vi "setUp.vi"(8 "error in (no error)":errorcluster, 11 "reference in":refnum<class "Test TCP Stream Disconnect.lvclass">) -> (0 "error out":errorcluster, 3 "reference out":refnum<class "Test TCP Stream Disconnect.lvclass">)   [LabVIEW 2020, in "Test TCP Stream Disconnect.lvclass"]
doc: "setUp runs prior to the test method during test execution. Use this method to initialize any object data required by your tests."
uses:
  Test TCP Stream Disconnect.lvclass
  <vilib>/addons/_JKI Toolkits/VI Tester/TestCase.llb/TestCase.lvclass
  Source/Protocols/TCP Strategy/TCP Stream Initiator/TCP Stream Initiator.lvclass
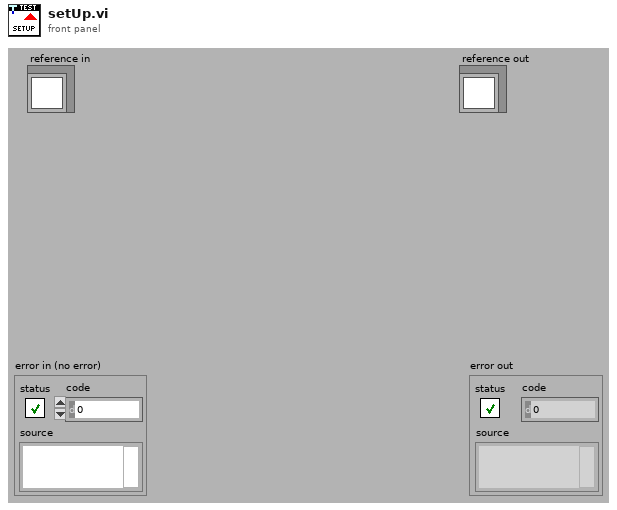
[diagram p1: front panel]
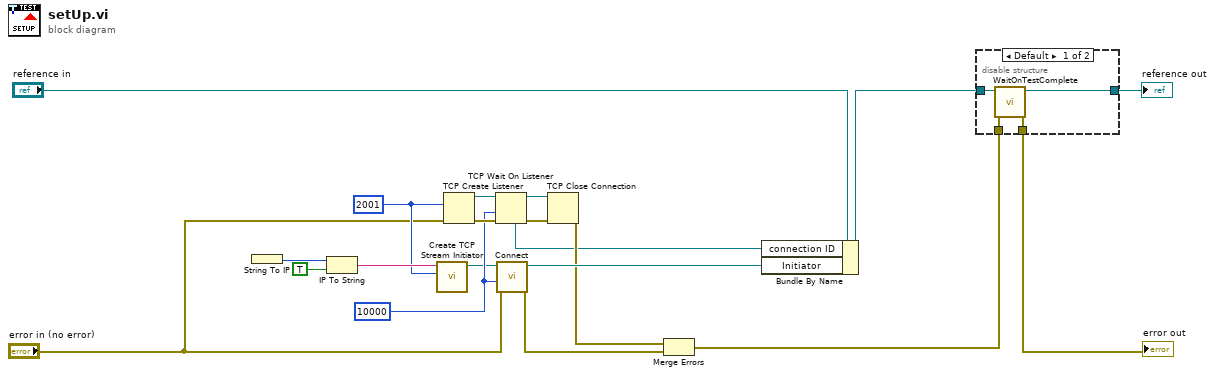
[diagram p0: block diagram]
diagram:
  w7 = u16 2001 ("port")
  w12 = 10000 ("timeout")
  n1 = String To IP() -> (0:w10:u32)  [unwired: 1 in]
  n2 = IP To String(1:TRUE ("dot notation? (F)"), 2:w10) -> (0:w9:string)
  n3 = call "Create TCP Stream Initiator.vi"("Remote Port"=w7, "Remote Address"=w9) -> ("TCP Stream Initiator"=w8:refnum<class "TCP Stream Initiator.lvclass">)  [unwired: 9 in]
  n4 = TCP Create Listener(8:"error in (no error)", 10:w7) -> (0:w16:errorcluster, 3:w15:refnum<k5>)  [unwired: 3 in, 1 out]
  n5 = TCP Wait On Listener(8:w16, 9:w12, 11:w15) -> (0:w14:errorcluster, 3:w13:refnum<k5>, 4:w1:refnum<k5>)  [unwired: 1 in, 2 out]
  n6 = call-dynamic "Connect.vi"("error in (no error)"="error in (no error)", "timeout"=w12, "TCP Stream Initiator in"=w8) -> ("error out"=w3:errorcluster, "TCP Stream Initiator out"=w6:refnum<class "TCP Stream Initiator.lvclass">)  [unwired: 7 in]
  n7 = TCP Close Connection(connection ID=w13, error in (no error)=w14) -> (error out=w2:errorcluster)  [unwired: 1 in, 1 out]
  n8 = Merge Errors(w2, w3) -> (w4:errorcluster)
  n9 = Bundle By Name(cluster="reference in", "connection ID"=w1, "Initiator"=w6) -> (w17:refnum<class "Test TCP Stream Disconnect.lvclass">)
  n10 = disable-structure shown="Default" {
    disable-tunnel: w4 -> [w24 w25]
    disable-tunnel: [w23 w25] -> w20
    disable-tunnel: [w22 w26] -> w18
    disable-tunnel: w17 -> [w21 w26]
    frame condition #0 (active) {
      n11 = call <vilib>:"WaitOnTestComplete.vi"("error in (no error)"=w24, "TestCase in"=w21) -> ("error out"=w23:errorcluster, "TestCase out"=w22:refnum<class "Test TCP Stream Disconnect.lvclass">)  [unwired: 8 in]
    }
    frame condition #1 {
    }
  }
  "error out" <- w20
  "reference out" <- w18
